vi "Apply Previous Amplitude.vi"(8 "error in (no error)":errorcluster, 10 "waveform in":waveform(dbl), 11 "SV Signal in":refnum<class "SV Signal.lvclass">) -> (0 "error out":errorcluster, 2 "waveform out":waveform(dbl), 3 "SV Signal out":refnum<class "SV Signal.lvclass">)   [LabVIEW 2017, in "SV Signal.lvclass"]
uses:
  <vilib>/addons/_NISVFA/_Generation/Signal Generation/SV Signal/SV Signal.lvclass
  <vilib>/addons/_NISVFA/_Generation/Signal Generation/SV Signal/SV Signal.lvclass/SV Signal.ctl
  <vilib>/addons/_NISVFA/_Generation/Signal Generation/SV Signal/sv_Signal State Attribute.ctl
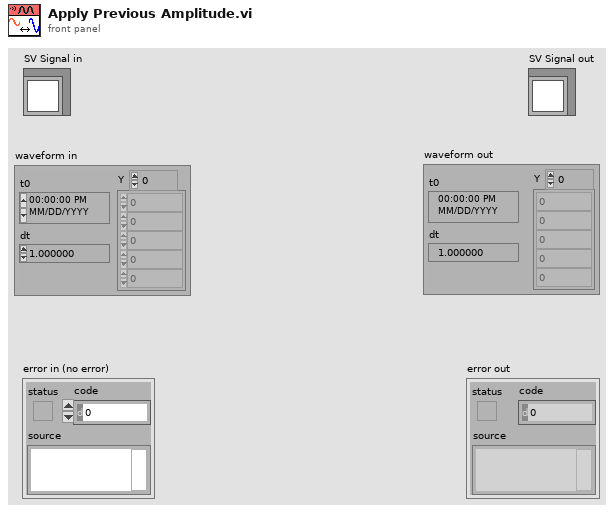
[diagram p1: front panel]
types:
  T1 = typedef "SV Signal.lvclass/sv_Signal State Attribute.ctl" = string
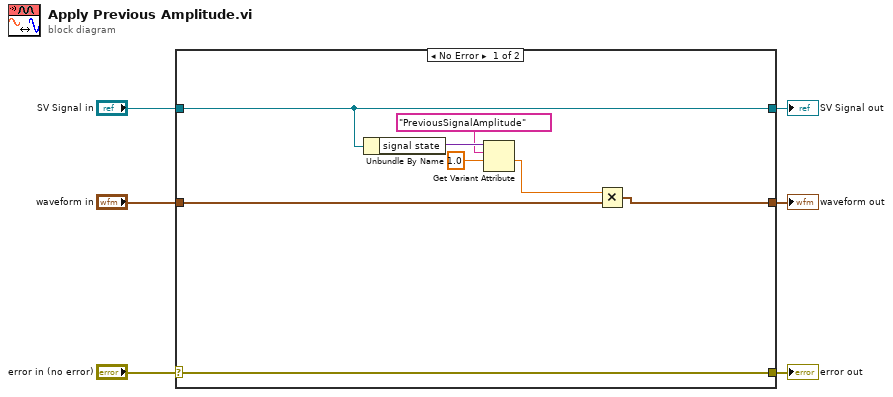
[diagram p0: block diagram]
diagram:
  n1 = case shown="No Error" "error in (no error)" {
    selector: "error in (no error)" -> [w14 w17]
    tunnel: [w14 w17] -> w5
    tunnel: [w10 w16] -> w3
    tunnel: "SV Signal in" -> [w10 w16]
    tunnel: "waveform in" -> [w8 w15]
    tunnel: [w7 w15] -> w1
    frame No Error {
      n2 = Unbundle By Name(w10) -> ("signal state"=w13:variant)
      n3 = Get Variant Attribute(Variant=w13, name=T1 "PreviousSignalAmplitude" ("attribute"), default value (empty Variant)=1.0) -> (value=w9:dbl)  [unwired: 1 in, 3 out]
      n4 = Multiply(x=w9, y=w8) -> (x*y=w7:waveform(dbl))
    }
    frame Error {
    }
  }
  "error out" <- w5
  "SV Signal out" <- w3
  "waveform out" <- w1
